vi "initialize hardware.vi"(7 "Reset (False)":bool, 8 "error in (no error)":errorcluster, 9 "devport":string, 10 "Settings":T1={"devport"="", "Position"={"Axis 1"={"Value"=0.0, "Min"=0.0, "Max"=0.0, "StepSize"=0.0, "Tolerance"=0.0, "ValueActual"=0.0}, "Axis 2"={"Value"=0.0, "Min"=0.0, "Max"=0.0, "StepSize"=0.0, "Tolerance"=0.0, "ValueActual"=0.0}, "Axis 3"={"Value"=0.0, "Min"=0.0, "Max"=0.0, "StepSize"=0.0, "Tolerance"=0.0, "ValueActual"=0.0}}, "Power"={"Axis 1"=enum."off", "Axis 2"=enum."off", "Axis 3"=enum."off"}, "Status"={"Axis 1"=enum."Not referenced", "Axis 2"=enum."Not referenced", "Axis 3"=enum."Not referenced"}, "Backlash"={"Axis 1"={"Value"=0.0, "Min"=0.0, "Max"=0.0, "StepSize"=0.0, "Tolerance"=0.0, "ValueActual"=0.0}, "Axis 2"={"Value"=0.0, "Min"=0.0, "Max"=0.0, "StepSize"=0.0, "Tolerance"=0.0, "ValueActual"=0.0}, "Axis 3"={"Value"=0.0, "Min"=0.0, "Max"=0.0, "StepSize"=0.0, "Tolerance"=0.0, "ValueActual"=0.0}}, "Home"={"Axis 1"={"Value"=0.0, "Min"=0.0, "Max"=0.0, "StepSize"=0.0, "Tolerance"=0.0, "ValueActual"=0.0}, "Axis 2"={"Value"=0.0, "Min"=0.0, "Max"=0.0, "StepSize"=0.0, "Tolerance"=0.0, "ValueActual"=0.0}, "Axis 3"={"Value"=0.0, "Min"=0.0, "Max"=0.0, "StepSize"=0.0, "Tolerance"=0.0, "ValueActual"=0.0}}, "MoveToHardLimit"={"Axis 1"=enum."pos", "Axis 2"=enum."pos", "Axis 3"=enum."pos"}, "relativeMove"={"Axis 1neg"=enum."off", "Axis 2neg"=enum."off", "Axis 3neg"=enum."off", "Axis 1pos"=enum."off", "Axis 2pos"=enum."off", "Axis 3pos"=enum."off"}, "stepsize"={"Value"=0.0, "Min"=0.0, "Max"=0.0, "StepSize"=0.0, "Tolerance"=0.0, "ValueActual"=0.0}, "automotoroff"=enum."off", "ResetBeforeMove"=enum."off", "Enable"={"Axis 1"=enum."on", "Axis 2"=enum."on", "Axis 3"=enum."on"}}, 11 "ESP302 in":refnum<class "ESP302.lvclass">) -> (0 "error out":errorcluster, 2 "VISA resource name out":refnum<visa-resource-name>, 3 "ESP302 out":refnum<class "ESP302.lvclass">)   [LabVIEW 2020, in "ESP302.lvclass"]
uses:
  ESP302.lvclass
  SettingsTypdef.ctl
  shared/OnOffTypeDef.ctl
  status_TypDef.ctl
  Hardware limit.ctl
  shared/CompressAndUpdate(Poly)/CompressAndUpdate(Enum).vi
  shared/CompressAndUpdate(Poly)/CompressAndUpdate(Numeric).vi
  ESP301.lvclass
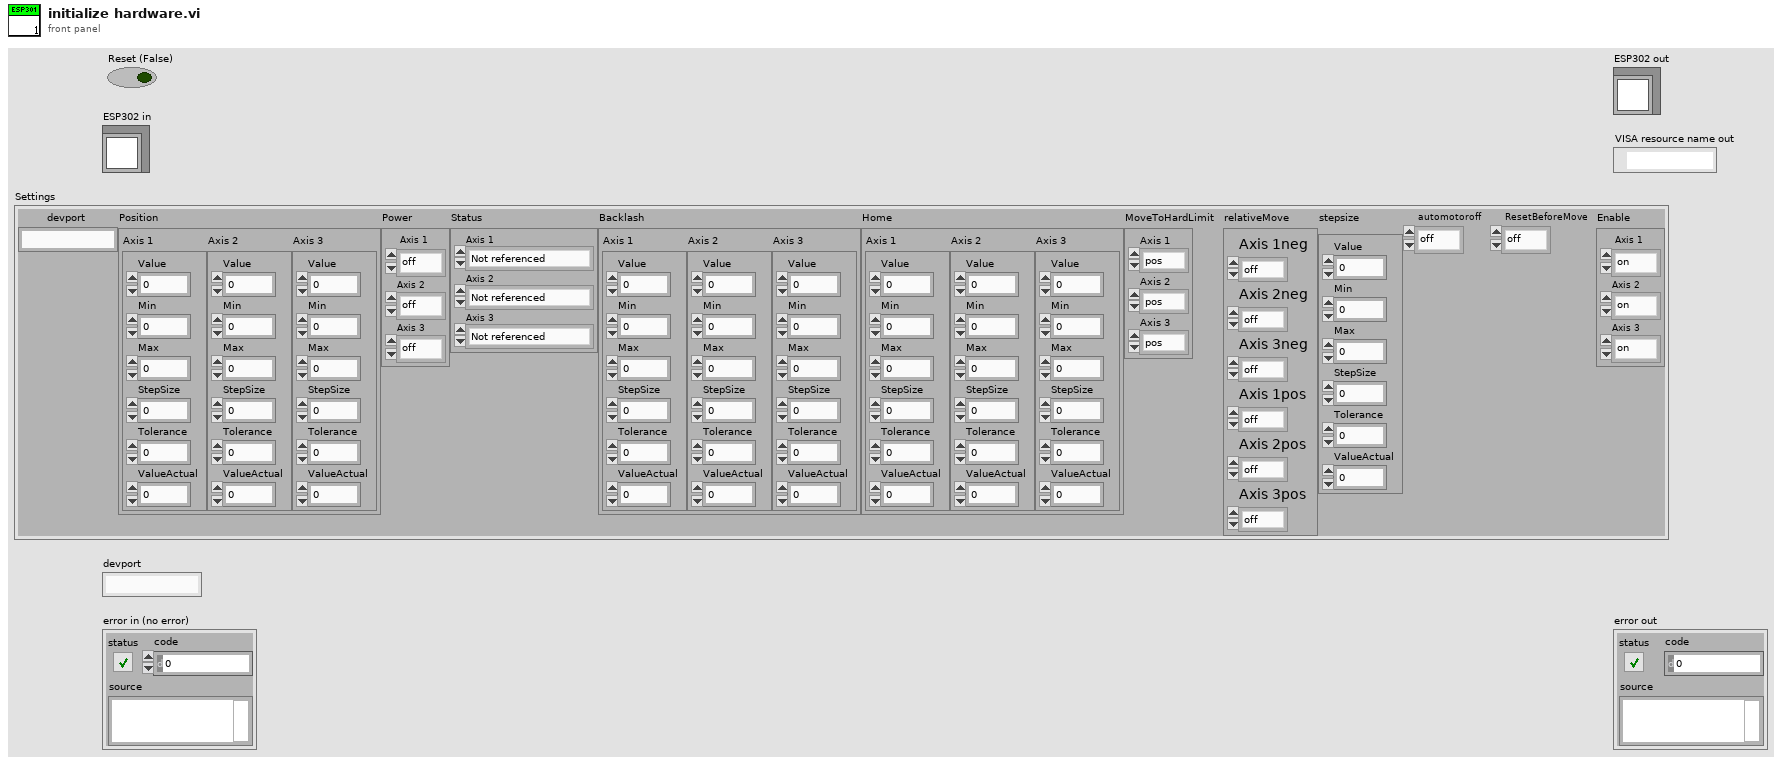
[diagram p1: front panel]
types:
  T1 = typedef "ESP301.lvclass/SettingsTypdef.ctl" = cluster{"devport":string, "Position":cluster{"Axis 1":cluster{"Value":dbl, "Min":dbl, "Max":dbl, "StepSize":dbl, "Tolerance":dbl, "ValueActual":dbl}, "Axis 2":cluster{"Value":dbl, "Min":dbl, "Max":dbl, "StepSize":dbl, "Tolerance":dbl, "ValueActual":dbl}, "Axis 3":cluster{"Value":dbl, "Min":dbl, "Max":dbl, "StepSize":dbl, "Tolerance":dbl, "ValueActual":dbl}}, "Power":cluster{"Axis 1":T2, "Axis 2":T2, "Axis 3":T2}, "Status":cluster{"Axis 1":T3, "Axis 2":T3, "Axis 3":T3}, "Backlash":cluster{"Axis 1":cluster{"Value":dbl, "Min":dbl, "Max":dbl, "StepSize":dbl, "Tolerance":dbl, "ValueActual":dbl}, "Axis 2":cluster{"Value":dbl, "Min":dbl, "Max":dbl, "StepSize":dbl, "Tolerance":dbl, "ValueActual":dbl}, "Axis 3":cluster{"Value":dbl, "Min":dbl, "Max":dbl, "StepSize":dbl, "Tolerance":dbl, "ValueActual":dbl}}, "Home":cluster{"Axis 1":cluster{"Value":dbl, "Min":dbl, "Max":dbl, "StepSize":dbl, "Tolerance":dbl, "ValueActual":dbl}, "Axis 2":cluster{"Value":dbl, "Min":dbl, "Max":dbl, "StepSize":dbl, "Tolerance":dbl, "ValueActual":dbl}, "Axis 3":cluster{"Value":dbl, "Min":dbl, "Max":dbl, "StepSize":dbl, "Tolerance":dbl, "ValueActual":dbl}}, "MoveToHardLimit":cluster{"Axis 1":T4, "Axis 2":T4, "Axis 3":T4}, "relativeMove":cluster{"Axis 1neg":T2, "Axis 2neg":T2, "Axis 3neg":T2, "Axis 1pos":T2, "Axis 2pos":T2, "Axis 3pos":T2}, "stepsize":cluster{"Value":dbl, "Min":dbl, "Max":dbl, "StepSize":dbl, "Tolerance":dbl, "ValueActual":dbl}, "automotoroff":T2, "ResetBeforeMove":T2, "Enable":cluster{"Axis 1":T2, "Axis 2":T2, "Axis 3":T2}}
  T2 = typedef "OnOffTypeDef.ctl" = enum16{"off", "on"}
  T3 = typedef "status_TypDef.ctl" = enum16{"Not referenced", "Homing", "Moving", "Ready"}
  T4 = typedef "Hardware limit.ctl" = enum16{"pos", "neg"}
  T5 = cluster{"Axis 1":cluster{"Value":dbl, "Min":dbl, "Max":dbl, "StepSize":dbl, "Tolerance":dbl, "ValueActual":dbl}, "Axis 2":cluster{"Value":dbl, "Min":dbl, "Max":dbl, "StepSize":dbl, "Tolerance":dbl, "ValueActual":dbl}, "Axis 3":cluster{"Value":dbl, "Min":dbl, "Max":dbl, "StepSize":dbl, "Tolerance":dbl, "ValueActual":dbl}}
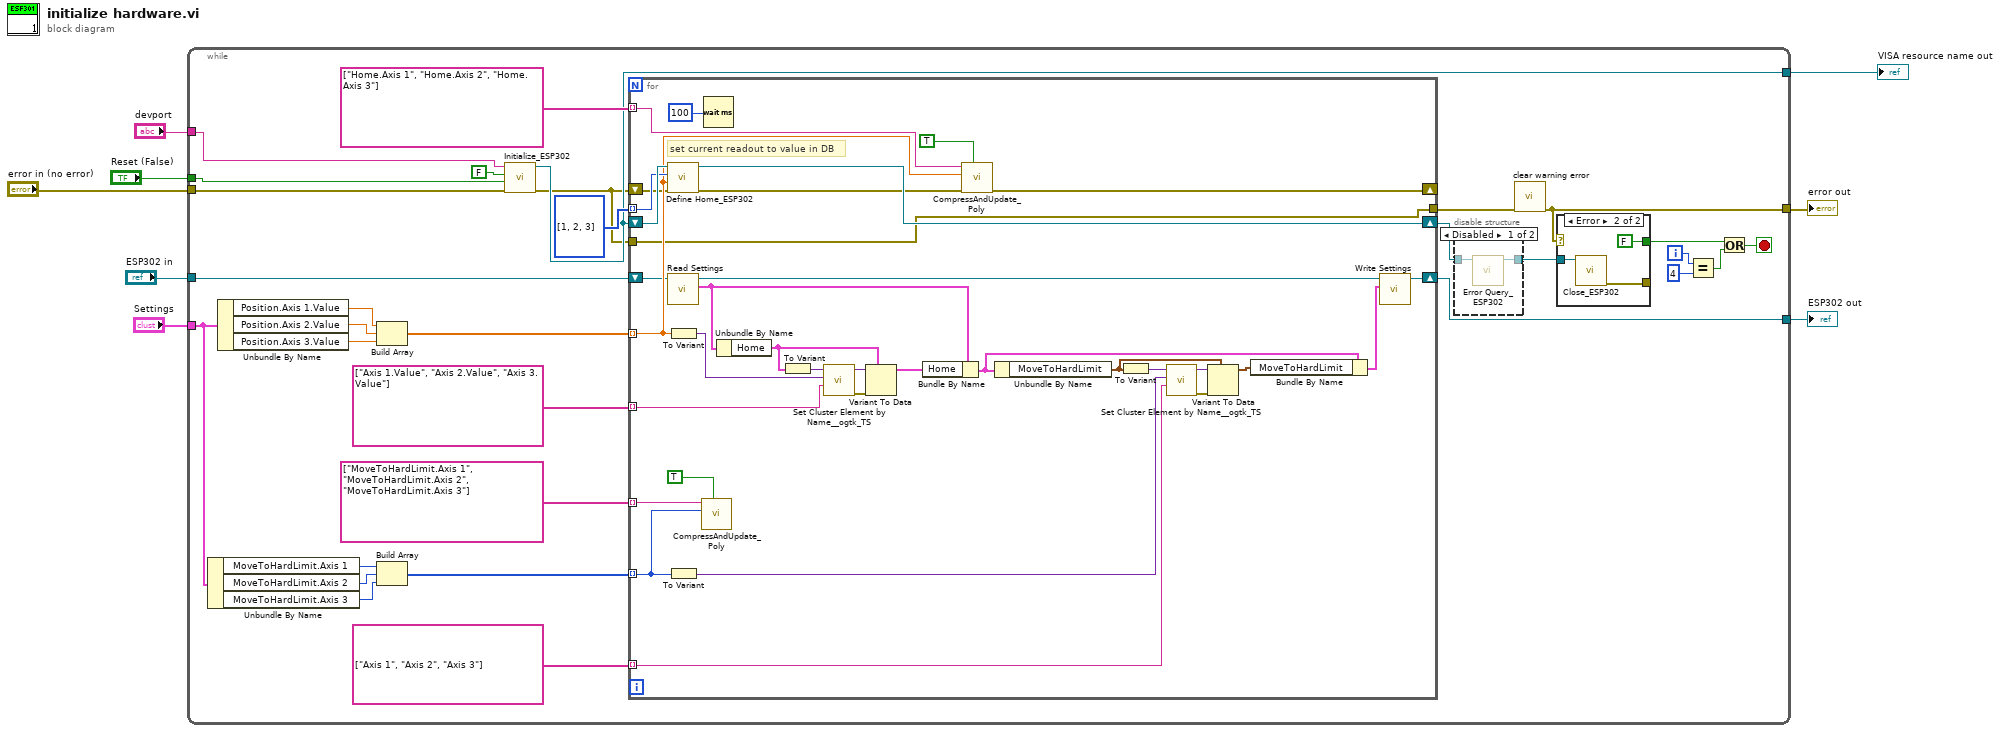
[diagram p0: block diagram]
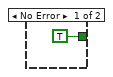
[diagram p3: hidden frame]
diagram:
  n1 = while {
    tunnel: "error in (no error)" -> [w39]
    tunnel: "devport" -> [w37]
    tunnel: "ESP302 in" -> [w9]
    tunnel: [w31] -> w4
    tunnel: [w21] -> w5
    tunnel: "Settings" -> [w20]
    tunnel: [w14] -> w7
    tunnel: "Reset (False)" -> [w10]
    i -> [w19]
    stop <- w16 stop-if-true
    n2 = Unbundle By Name(w20) -> ("MoveToHardLimit.Axis 1"=w24:T4, "MoveToHardLimit.Axis 2"=w25:T4, "MoveToHardLimit.Axis 3"=w26:T4)
    n3 = Unbundle By Name(w20) -> ("Position.Axis 1.Value"=w35:dbl, "Position.Axis 2.Value"=w34:dbl, "Position.Axis 3.Value"=w33:dbl)
    n4 = Build Array(w35, w34, w33) -> (w32:dbl[])
    n5 = Build Array(w24, w25, w26) -> (w23:T4[])
    n6 = call "Initialize_ESP302.vi"("VISA resource name"=w37, "ID Query (True)"=FALSE, "Reset (False)"=w10, "error in (no error)"=w39) -> ("VISA resource name out"=w21:refnum<visa-resource-name>, "error out"=w12:errorcluster)  [unwired: 5 in]
    n7 = for {
      shift-right: [w72] -> w28
      shift-left: w21 -> [w73]
      tunnel: i32[] [1, 2, 3] -> [w71] mode=indexing
      tunnel: w32 -> [w70] mode=indexing
      shift-right: [w47] -> w31
      shift-left: w9 -> [w51]
      tunnel: string[] ["Axis 1.Value", "Axis 2.Value", "Axis 3.Value"] ("set following Variables (empty = all avriables)") -> [w76] mode=indexing
      tunnel: string[] ["Home.Axis 1", "Home.Axis 2", "Home.Axis 3"] ("set following Variables (empty = all avriables)") -> [w74] mode=indexing
      shift-right: [w67] -> _
      shift-left: w12 -> [w69]
      tunnel: string[] ["MoveToHardLimit.Axis 1", "MoveToHardLimit.Axis 2", "MoveToHardLimit.Axis 3"] ("set following Variables (empty = all avriables)") -> [w65] mode=indexing
      tunnel: w23 -> [w59] mode=indexing
      tunnel: string[] ["Axis 1", "Axis 2", "Axis 3"] ("set following Variables (empty = all avriables)") -> [w58] mode=indexing
      tunnel: w12 -> [w56]
      tunnel: [w56] -> w11
      # "set current readout to value in DB"
      n8 = call "Define Home_ESP302.vi"("error in (no error)"=w69, "Home Position (0 units)"=w70, "Axis (1)"=w71, "VISA resource name"=w73) -> ("error out"=w68:errorcluster, "VISA resource name out"=w72:refnum<visa-resource-name>)  [unwired: 2 in]
      n9 = call-dynamic "Read Settings.vi"("ESP301 in"=w51) -> ("Settings"=w50:T1, "ESP301 out"=w49:refnum<class "ESP302.lvclass">)  [unwired: 8 in, 1 out]
      n10 = To Variant(anything=w70) -> (Variant=w53:variant)
      n11 = To Variant(anything=w59) -> (Variant=w54:variant)
      n12 = call-poly "CompressAndUpdate_Poly.vi"("force CVT update (false)"=TRUE ("force CVT update"), "enum variant"=w59, "command or variable name"=w65) -> ()  [unwired: 8 in, 1 out]
      n13 = Wait (ms)(milliseconds to wait=u32 100) -> ()  [unwired: 1 out]
      n14 = Unbundle By Name(w50) -> ("Home"=w79:T5)
      n15 = To Variant(anything=w79) -> (Variant=w52:variant)
      n16 = call "Set Cluster Element by Name__ogtk_TS.vi"("Element Name (\"\": New Element Data Name)"=w76, "New Element Value"=w53, "Cluster"=w52) -> ("error out"=w77:errorcluster, "VCluster out"=w78:variant)  [unwired: 6 in, 1 out]
      n17 = Variant To Data(error in=w77, type=w79, Variant=w78) -> (data=w80:T5)  [unwired: 1 out]
      n18 = Bundle By Name(cluster=w50, "Home"=w80) -> (w60:T1)
      n19 = call-poly "CompressAndUpdate_Poly.vi"("force CVT update (false)"=TRUE ("force CVT update"), "error in"=w68, "Numeric"=w70, "command or variable name"=w74) -> ("error out"=w67:errorcluster)  [unwired: 7 in]
      n20 = Unbundle By Name(w60) -> ("MoveToHardLimit"=w62:cluster{"Axis 1":T4, "Axis 2":T4, "Axis 3":T4})
      n21 = To Variant(anything=w62) -> (Variant=w55:variant)
      n22 = call "Set Cluster Element by Name__ogtk_TS.vi"("Element Name (\"\": New Element Data Name)"=w58, "New Element Value"=w54, "Cluster"=w55) -> ("error out"=w64:errorcluster, "VCluster out"=w63:variant)  [unwired: 6 in, 1 out]
      n23 = Variant To Data(error in=w64, type=w62, Variant=w63) -> (data=w61:cluster{"Axis 1":T4, "Axis 2":T4, "Axis 3":T4})  [unwired: 1 out]
      n24 = Bundle By Name(cluster=w60, "MoveToHardLimit"=w61) -> (w48:T1)
      n25 = call-dynamic "Write Settings.vi"("Settings"=w48, "ESP301 in"=w49) -> ("ESP301 out"=w47:refnum<class "ESP302.lvclass">)  [unwired: 8 in, 1 out]
    }
    n26 = disable-structure shown="Disabled" {
      disable-tunnel: w28 -> [w41 w42]
      disable-tunnel: [w40 w42] -> w15
      frame Disabled {
        n27 = call "Error Query_ESP302.vi"("VISA resource name"=w41) -> ("VISA resource name out"=w40:refnum<visa-resource-name>)  [unwired: 3 in, 3 out]
      }
      frame Enabled {
      }
    }
    n28 = call "clear warning error.vi"("error in"=w11) -> ("error out"=w14:errorcluster)  [unwired: 10 in]
    n29 = case shown="Error" w14 {
      tunnel: w15 -> [_ w45]
      tunnel: [TRUE FALSE] -> w13
      tunnel: [_ w44] -> _
      frame No Error {
      }
      frame Error {
        n30 = call "Close_ESP302.vi"("VISA resource name"=w45) -> ("error out"=w44:errorcluster)  [unwired: 10 in]
      }
    }
    n31 = Equal?(x=w19, y=4) -> (x = y?=w17:bool)
    n32 = Or(x=w13, y=w17) -> (x .or. y?=w16:bool)
  }
  "error out" <- w7
  "VISA resource name out" <- w5
  "ESP302 out" <- w4
